vi "SetAutoapproach.vi"(8 "error in":T5, 11 "Autoapproach Cluster":T1={"Delay"=-inf, "Threshold [a.u.]"=-inf, "Stop Condition"=-2147483648, "Speed"=-inf, "Steps / Approach"=-2147483648, "Approach Mode"=-2147483648, "Target Mode"=-2147483648} {"Target Mode" items=["[read only]"=-2147483648, "Loop On"=0, "Retract"=1, "Loop Off"=2]; "Approach Mode" items=["[read only]"=-2147483648, "Ramp"=0, "Loop"=1]; "Speed" format="%#_g V/s"; "Stop Condition" items=["[read only]"=-2147483648, "> Threshold"=0, "< Threshold"=1]; "Delay" format="%#_g ms"}) -> (0 "error out":T5, 3 "Autoapproach Output":T1={"Delay"=-inf, "Threshold [a.u.]"=-inf, "Stop Condition"=-2147483648, "Speed"=-inf, "Steps / Approach"=-2147483648, "Approach Mode"=-2147483648, "Target Mode"=-2147483648} {"Target Mode" items=["[read only]"=-2147483648, "Loop On"=0, "Retract"=1, "Loop Off"=2]; "Approach Mode" items=["[read only]"=-2147483648, "Ramp"=0, "Loop"=1]; "Speed" format="%#_g V/s"; "Stop Condition" items=["[read only]"=-2147483648, "> Threshold"=0, "< Threshold"=1]; "Delay" format="%#_g ms"})   [LabVIEW 2016]
doc: "Configures the auto approach functionality. The cluster contains:\n\n- Delay (float) [0 to 100000]\n- Threshold in mV, deg or Hz depending on input signal from Z Control (float) [without restraint]\n- Stop Condition (integer) [0 -- > Threshold; 1 -- < Threshold]\n- Speed in V/s (float) [0.0005 to 1000]\n- Steps per Approach (integer) [0 to 100]\n- Approach Mode (integer) [0 -- ramp; 1 -- loop]\n- Target Mode (integer) [0 -- loop on; 1-- retract; 2 -- loop off]\nBy passing -Inf (float) or -2147483648 (integer) as input values, the corresponding parameter(s) will be read out."
uses:
  Controls/Autoapproach_Parameters.ctl
  Controls/Stop-Condition-Autoapproach_Selection.ctl
  Controls/Autoapproach-Approach-Mode_Selection.ctl
  Controls/Autoapproach-Target-Mode_Selection.ctl
  Controls/Error_Out.ctl
  Files_ASC500/DLL/ASC500_RemoteControlV27.dll
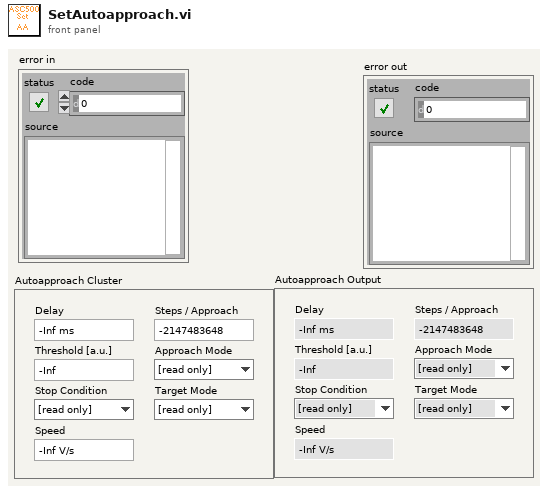
[diagram p1: front panel]
types:
  T1 = typedef "Autoapproach_Parameters.ctl" = cluster{"Delay":sgl, "Threshold [a.u.]":sgl, "Stop Condition":T2, "Speed":sgl, "Steps / Approach":i32, "Approach Mode":T3, "Target Mode":T4}
  T2 = typedef "Stop-Condition-Autoapproach_Selection.ctl" = i32
  T3 = typedef "Autoapproach-Approach-Mode_Selection.ctl" = i32
  T4 = typedef "Autoapproach-Target-Mode_Selection.ctl" = i32
  T5 = typedef "Error_Out.ctl" = errorcluster
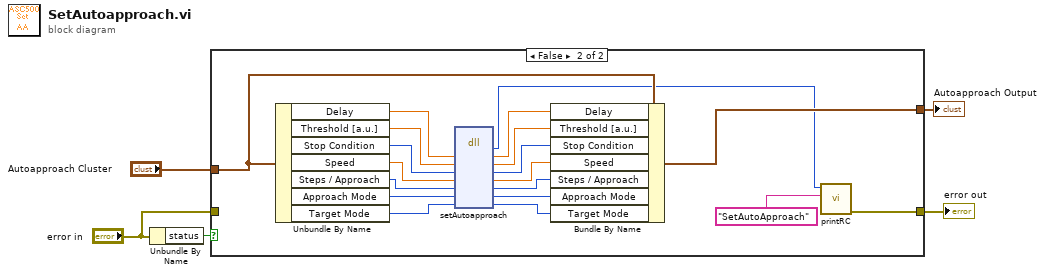
[diagram p0: block diagram]
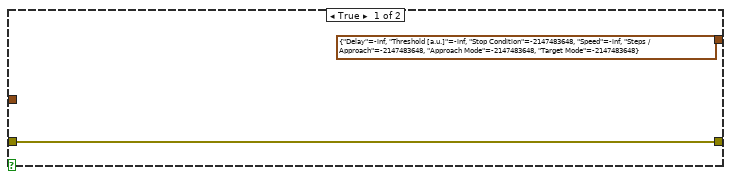
[diagram p2: hidden frame]
diagram:
  n1 = Unbundle By Name("error in") -> ("status"=w5:bool)
  n2 = case shown="False" w5 {
    tunnel: [w6 w11] -> w4
    tunnel: "Autoapproach Cluster" -> [_ w14]
    tunnel: [T1 {"Delay"=-inf, "Threshold [a.u.]"=-inf, "Stop Condition"=-2147483648, "Speed"=-inf, "Steps / Approach"=-2147483648, "Approach Mode"=-2147483648, "Target Mode"=-2147483648} ("Autoapproach Cluster") w13] -> w1
    tunnel: "error in" -> [w6 _]
    frame True {
    }
    frame False {
      n3 = Unbundle By Name(w14) -> ("Delay"=w26:sgl, "Threshold [a.u.]"=w25:sgl, "Stop Condition"=w24:T2, "Speed"=w23:sgl, "Steps / Approach"=w22:i32, "Approach Mode"=w21:T3, "Target Mode"=w20:T4)
      n4 = dll-call lib="G:/SCMOperations/Share/ELE/Produkt Information/ASC500/04 Remote Control/02 development versions/2018Nov06/Files_ASC500/DLL/ASC500_RemoteControlV27.dll" fn="setAutoapproach"("Delay"=w26, "Threshold"=w25, "Stop Condition"=w24, "Speed"=w23, "Steps / Approach"=w22, "Approach Mode"=w21, "Target Mode"=w20) -> ("return type"=w8:i32, "Delay"=w9:sgl, "Threshold"=w19:sgl, "Stop Condition"=w18:i32, "Speed"=w17:sgl, "Steps / Approach"=w16:i32, "Approach Mode"=w12:i32, "Target Mode"=w15:i32)  [unwired: 3 in, 2 out]
      n5 = Bundle By Name(cluster=w14, "Delay"=w9, "Threshold [a.u.]"=w19, "Stop Condition"=w18, "Speed"=w17, "Steps / Approach"=w16, "Approach Mode"=w12, "Target Mode"=w15) -> (w13:T1)
      n6 = call "printRC.vi"("additional information"="SetAutoApproach", "RC"=w8) -> ("error out"=w11:T5)  [unwired: 9 in]
    }
  }
  "error out" <- w4
  "Autoapproach Output" <- w1
